vi "get-tag-by-id.vi"(8 "error in (no error)":errorcluster, 9 "id":u32, 11 "CANtable in":refnum<class "bAPPdata.lvclass">) -> (0 "error out":errorcluster, 1 "tag":string, 3 "CANtable out":refnum<class "bAPPdata.lvclass">)   [LabVIEW 2015, in "bAPPdata.lvclass"]
uses:
  bAPPdata.lvclass
  bAPPdata.lvclass/bAPPdata.ctl
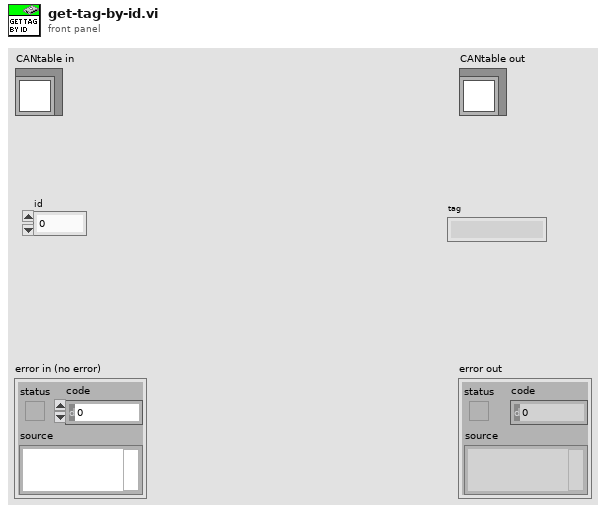
[diagram p1: front panel]
types:
  T1 = typedef "bAPPdata.lvclass/table-data.ctl" = T2[]
  T2 = typedef "bAPPdata.lvclass/table-contents.ctl" = cluster{"id":u32, "tag":string, "frame.type":T3, "last.frame":T4, "tMsgData":T6, "child.tags":string[], "bit-payload":bool[]}
  T3 = typedef "frame.type.ctl" = enum16{"FRAME NOT DEFINED", "DUT OUTPUT FRAME", "DUT INPUT FRAME"}
  T4 = typedef "XNET Frame CAN.ctl" = cluster{"timestamp":timestamp, "payload":u8[], "identifier":u32, "type":T5, "extended?":bool, "echo?":bool}
  T5 = typedef "XNET Frame Type CAN.ctl" = u8
  T6 = typedef "nMsgData.ctl" = cluster{"dwID":u32, "count":u32, "dwCycleTime":dbl, "dwTime":dbl, "new msg":bool}
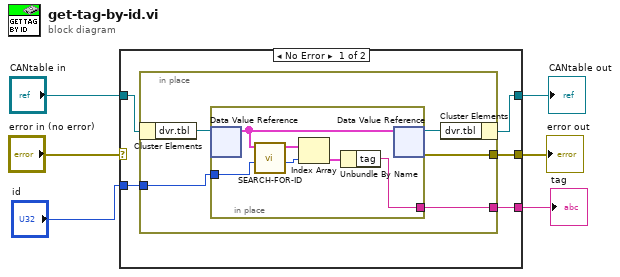
[diagram p0: block diagram]
diagram:
  n1 = case shown="No Error" "error in (no error)" {
    selector: "error in (no error)" -> [_ w24]
    tunnel: [w7 w24] -> w5
    tunnel: [w10 w23] -> w3
    tunnel: "CANtable in" -> [w11 w23]
    tunnel: "id" -> [w9 _]
    tunnel: [w8 _] -> w1
    frame No Error {
      n2 = in-place {
        in-place-border: w9 -> [w14]
        in-place-border: [w13] -> w8
        in-place-border: [w12] -> w7
        n3 = in-place-cluster #1(w11) -> ("dvr.tbl"=w16:refnum<data-value>)
        n4 = in-place {
          in-place-border: w14 -> [w22]
          in-place-border: [w18] -> w13
          n5 = in-place-dvr #2(w16) -> (w21:T1)  [unwired: 1 out]
          n6 = call "SEARCH-FOR-ID.vi"("ID"=w22, "tbl.list"=w21) -> ("idx"=w20:i32, "tbl.list out"=w17:T2[])  [unwired: 8 in]
          n7 = Index Array(array=w17, index=w20) -> (element=w19:T2)
          n8 = Unbundle By Name(w19) -> ("tag"=w18:string)
          n9 = in-place-dvr #2(w21) -> (w15:refnum<data-value>, w12:errorcluster)
        }
        n10 = in-place-cluster #1("dvr.tbl"=w15) -> (w10:refnum<class "bAPPdata.lvclass">)
      }
    }
    frame Error {
    }
  }
  "error out" <- w5
  "CANtable out" <- w3
  "tag" <- w1
